vi "PH_Timing.PC Phase FEs.vi"(0 "i ref in":refnum<vi>, 2 "FE Phase":T1 {"Phase" format="%#_12p"}, 5 "error IO":errorcluster) -> (14 "i ref out":refnum<vi>, 19 "error out":errorcluster)   [LabVIEW 2014, in "PH_Timing.lvlib"]
doc: "This is a certain process case of Timing."
uses:
  PH_Timing.lvlib
  PH_Timing.Phase FEs.ctl
  PH_Devices/PH_SRDG645/PH_SRDG645.lvlib
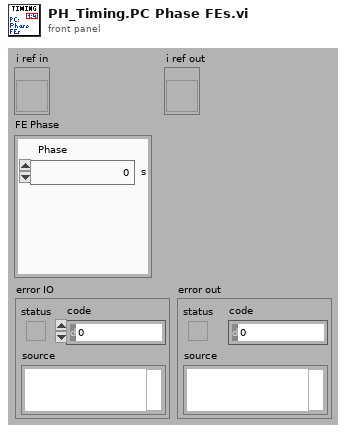
[diagram p1: front panel]
types:
  T1 = typedef "PH_Timing.lvlib/PH_Timing.Phase FEs.ctl" = cluster{"Phase":dbl}
  T2 = typedef "PH_Timing.lvlib/PH_Timing.i attribute.ctl" = cluster{"Sequencer":cluster{"linked?":bool, "Proc State":string, "Ref State":refnum<vi>}, "Gate Generator":cluster{"GD":cluster{"Device Status":T3, "linked?":bool}, "Settings":T4, "GUI Ref":refnum<vi>}, "Interlock Bypass":cluster{"Instancename":string, "Switch linked?":bool, "Device Status":T3, "Ref Status":refnum<vi>}, "Roughtuner":cluster{"Settings":T5, "GUI Ref":refnum<vi>, "GD":cluster{"Device Status":T3, "linked?":bool}}, "0,5Hz Gater":cluster{"Settings":T6, "GUI Ref":refnum<vi>, "GD":cluster{"Device Status":T3, "linked?":bool}}, "Slow Trigger":cluster{"Settings":T7, "GUI Ref":refnum<vi>, "Service ID Delay":i32, "Service ID Ext Trig":i32, "Wanted Settings":T7}, "Timing Mode":cluster{"Mode":T8, "GUI Ref":refnum<vi>, "Service ID T2":i32, "Service ID Mode":i32, "Wanted Mode":T8}, "ns Generator":cluster{"Settings":T9, "ns Generator Settings":refnum<vi>, "GD":cluster{"Device Status":T3, "linked?":bool}}, "Phase FEs":cluster{"Settings":T1, "GUI Ref":refnum<vi>, "Service ID Phase":i32, "Wanted Settings":T1}, "GD GUI Refs":refnum<vi>[], "Heads":T12[], "GUI Ref Delete":refnum<vi>}
  T3 = typedef "PH_StatusHandler.lvlib/PH_StatusHandler.Status.ctl" = i16
  T4 = typedef "PH_Timing.lvlib/PH_Timing.GateGen.ctl" = cluster{"Instance":string, "Channel Gate":i32, "Channel T2":i32, "Width Gate":dbl, "Width T2":dbl, "Delay Gate":dbl, "Delay T2":dbl, "Gate activ":bool, "T2 activ":bool, "System Mode":enum16{"Normal", "Single", "Burst", "Duty Cycle"}}
  T5 = typedef "PH_Timing.lvlib/PH_Timing.Roughtuner.ctl" = cluster{"Instance":string, "Phase PHELIX / UNILAC":cluster{"Channel":u16, "relative to":u16, "Delay [ms]":dbl}, "Pulse Length":cluster{"Channel":u16, "relative to":u16, "Delay [ms]":dbl}, "Trigger":cluster{"externally?":bool, "Rate [Hz]":dbl}}
  T6 = typedef "PH_Timing.lvlib/PH_Timing.0.5HzGater.ctl" = cluster{"Instance":string, "Channel ns FE Delay":i32, "Channel 0.5Hz":i32, "Width ns FE Delay":dbl, "Width 0.5Hz":dbl, "Delay ns FE Delay":dbl, "Delay 0.5Hz":dbl, "ns FE Delay active":bool, "0.5Hz activ":bool, "ns FE Delay inverted":bool, "0.5Hz inverted":bool}
  T7 = typedef "PH_Timing.lvlib/PH_Timing.Slow Trigger Settings.ctl" = cluster{"Delay":dbl, "externally triggered?":bool}
  T8 = typedef "PH_Timing.lvlib/PH_Timing.Timing Mode.ctl" = cluster{"T2":i16, "Modeselector":enum32{"10 Hz", "0.5 Hz", "Shot"}}
  T9 = typedef "PH_Timing.lvlib/PH_Timing.ns Generator.ctl" = cluster{"Instance":string, "Phase fs / ns FE":cluster{"Channel":T10, "Settings":T11}}
  T10 = typedef "Stanford Research DG645 - Driver.lvlib/Channel.ctl" = i32
  T11 = typedef "PH_SRDG645.lvlib/PH_SRDG645.Channel Settings.ctl" = cluster{"Delay [s]":dbl, "relative to":i32}
  T12 = typedef "PH_Timing.lvlib/PH_Timing.PU Data.ctl" = cluster{"linked?":bool, "Data":T13, "GD":cluster{"Device Status":T3, "linked?":bool}, "GUI Ref":refnum<vi>, "PU":T14}
  T13 = typedef "PH_Timing.lvlib/PH_Timing.PU Info.ctl" = cluster{"Act CH?":bool, "GD":string, "CH":i32, "Delay":dbl, "active":bool, "in Use?":bool}
  T14 = typedef "PH_PP_Common.lvlib/PH_PP_Common.PUs.ctl" = enum16{"no Info", "PA-19mm-1", "PA-19mm-2", "PA-45mm-PILC", "PA-45mm-MAIN", "MA-PU-1", "MA-PU-2", "MA-PU-3", "MA-PU-4", "MA-PU-5", "MA-PU-6", "MA-FR", "MA-PILC", "PA-45mm-DP"}
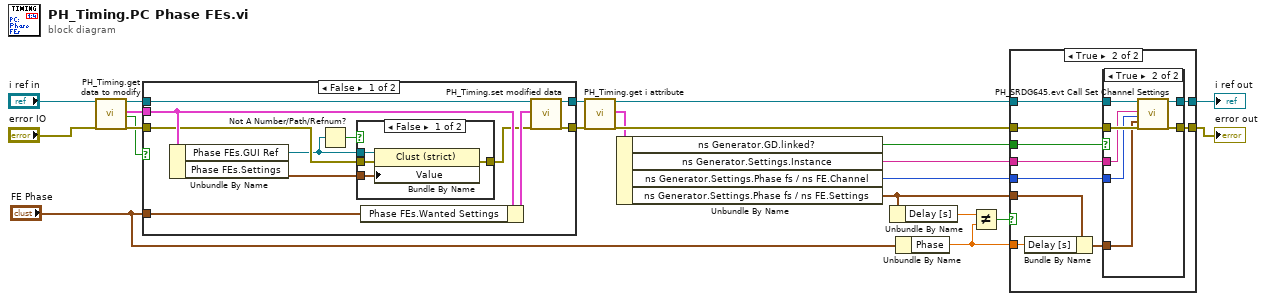
[diagram p0: block diagram]
diagram:
  n1 = call "PH_Timing.get data to modify.vi"("i ref in"="i ref in", "error in (no error)"="error IO") -> ("i ref out"=w19:refnum<vi>, "i attribute"=w17:T2, "timed out"=w16:bool, "error out"=w18:errorcluster)  [unwired: 14 in]
  n2 = case shown="False" w16 {
    tunnel: w19 -> [w32 w39]
    tunnel: [w31 w39] -> w12
    tunnel: w18 -> [w25 w38]
    tunnel: [w30 w38] -> w11
    tunnel: w17 -> [w27 _]
    tunnel: "FE Phase" -> [w28 _]
    frame False {
      n3 = Unbundle By Name(w27) -> ("Phase FEs.GUI Ref"=w22:refnum<vi>, "Phase FEs.Settings"=w26:T1)
      n4 = Not A Number/Path/Refnum?(number/path/refnum=w22) -> (NaN/Path/Refnum?=w23:bool)
      n5 = case shown="False" w23 {
        tunnel: w22 -> [w36 _]
        tunnel: w26 -> [w35 _]
        tunnel: w25 -> [w34 w37]
        tunnel: [w33 w37] -> w24
        frame False {
          n6 = property class="Clust (strict)"(reference=w36, error in=w34, "Value"=w35) -> (error out=w33:errorcluster)  [unwired: 1 out]
        }
        frame True {
        }
      }
      n7 = Bundle By Name(cluster=w27, "Phase FEs.Wanted Settings"=w28) -> (w29:T2)
      n8 = call "PH_Timing.set modified data.vi"("i ref in"=w32, "i attribute"=w29, "error in (no error)"=w24) -> ("i ref out"=w31:refnum<vi>, "error out"=w30:errorcluster)  [unwired: 15 in]
    }
    frame True {
    }
  }
  n9 = call "PH_Timing.get i attribute.vi"("i ref in"=w12, "error in (no error)"=w11) -> ("i ref out"=w14:refnum<vi>, "i attribute"=w13:T2, "error out"=w15:errorcluster)  [unwired: 15 in]
  n10 = Unbundle By Name(w13) -> ("ns Generator.GD.linked?"=w1:bool, "ns Generator.Settings.Instance"=w2:string, "ns Generator.Settings.Phase fs / ns FE.Channel"=w8:T10, "ns Generator.Settings.Phase fs / ns FE.Settings"=w6:T11)
  n11 = Unbundle By Name(w6) -> ("Delay [s]"=w5:dbl)
  n12 = Unbundle By Name("FE Phase") -> ("Phase"=w4:dbl)
  n13 = Not Equal?(x=w5, y=w4) -> (x != y?=w3:bool)
  n14 = case shown="True" w3 {
    tunnel: w15 -> [w40 w51]
    tunnel: w14 -> [w41 w50]
    tunnel: [w41 w49] -> w10
    tunnel: [w40 w48] -> w9
    tunnel: w8 -> [_ w47]
    tunnel: w6 -> [_ w46]
    tunnel: w4 -> [_ w44]
    tunnel: w2 -> [_ w43]
    tunnel: w1 -> [_ w42]
    frame False {
    }
    frame True {
      n15 = Bundle By Name(cluster=w46, "Delay [s]"=w44) -> (w45:T11)
      n16 = case shown="True" w42 {
        tunnel: w51 -> [w52 w59]
        tunnel: w50 -> [w53 w60]
        tunnel: [w52 w58] -> w48
        tunnel: [w53 w57] -> w49
        tunnel: w43 -> [_ w56]
        tunnel: w47 -> [_ w55]
        tunnel: w45 -> [_ w54]
        frame False {
        }
        frame True {
          n17 = call "PH_SRDG645.evt Call Set Channel Settings.vi"("i ref in"=w60, "Generator Instance"=w56, "Channel to set"=w55, "Channel Settings"=w54, "error IO"=w59) -> ("i ref out"=w57:refnum<vi>, "error out"=w58:errorcluster)  [unwired: 13 in]
        }
      }
    }
  }
  "error out" <- w9
  "i ref out" <- w10
